vi "Main.vi"() -> ()   [LabVIEW 2020]
uses:
  _lib/Root.lvlibp/Root.lvclass
  0c08c685-3369-46e5-9f6c-9a8c11b7282d.vi
  0c08c685-3369-46e5-9f6c-9a8c11b7282d.vi/a06a5617-693f-4e7a-880a-01e7210d5b34.vi
  0c08c685-3369-46e5-9f6c-9a8c11b7282d.vi/a86dd2ad-e02c-4951-b0d8-e9482f107a59.vi
  0c08c685-3369-46e5-9f6c-9a8c11b7282d.vi/2fe82b45-d63b-4374-a5d2-02a331a98b71.vi
  0c08c685-3369-46e5-9f6c-9a8c11b7282d.vi/09bee0a5-df0d-4391-90c9-116df187134d.vi
  0c08c685-3369-46e5-9f6c-9a8c11b7282d.vi/1c1c90a5-34b6-4f03-abf8-3ec97f905fca.vi
  0c08c685-3369-46e5-9f6c-9a8c11b7282d.vi/c25736fa-ea5e-462f-8a61-d5812afa17aa.vi
  <userlib>/_NEVSTOP/LabVIEW-ClassProviderShell/_Support/__File Exists - Scalar__ogtk.vi
  <userlib>/_NEVSTOP/LabVIEW-ClassProviderShell/_Support/__Strip Path Extension - String__ogtk.vi
  <vilib>/Utility/LVLibp/Get Exported File List.vi
  <vilib>/Utility/LVClass/Get LV Class Default Value.vi
  <userlib>/_NEVSTOP/LabVIEW-ClassProviderShell/_Support/__Wait(ms) If Input Valid.vi
  <vilib>/Utility/libraryn.llb/Recursive File List.vi
  <vilib>/Utility/libraryn.llb/Check if File or Folder Exists.vi
  <userlib>/_NEVSTOP/LabVIEW-ClassProviderShell/_Support/__Recursive File List with Exclude Option.vi
panel:
  out "result":dbl
  in  "b":dbl=20.0
  in  "a":dbl=100.0
  in  "Listbox":i32(listbox)
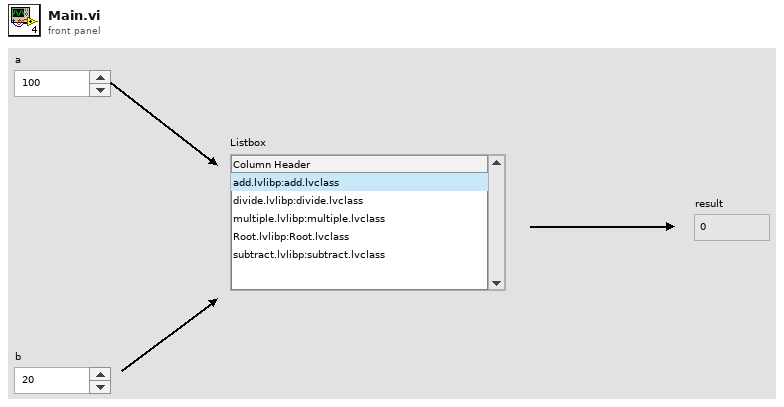
[diagram p1: front panel]
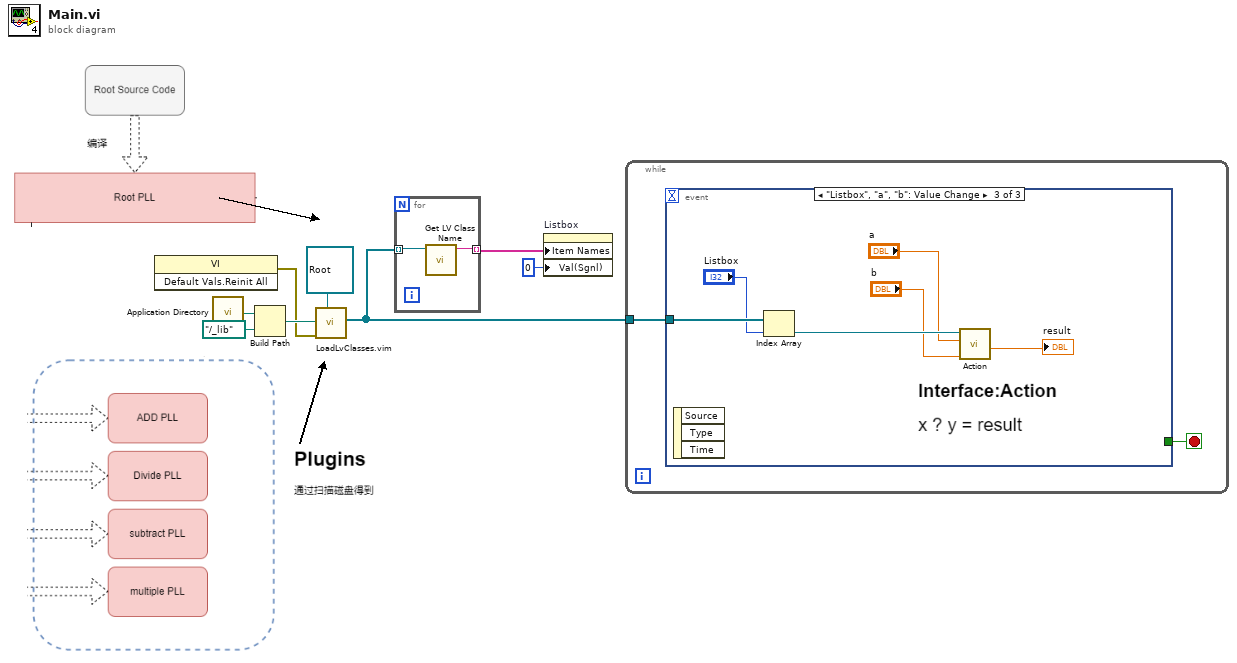
[diagram p0: block diagram]
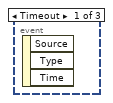
[diagram p2: hidden frame]
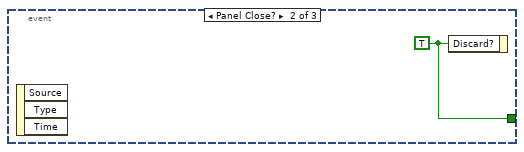
[diagram p3: hidden frame]
diagram:
  n1 = invoke class="VI" method="Default Vals.Reinit All"() -> (error out=w1:errorcluster)  [unwired: 3 in, 2 out]
  n2 = call <vilib>:"Application Directory.vi"() -> ("Application Directory"=w7:path)
  n3 = Build Path(base path=w7, name or relative path=path "../_lib") -> (appended path=w5:path)
  n4 = call "LoadLvClasses.vim"("ClassType"=refnum<class "Root.lvclass"> refnum ("Root.lvlibp:Root.lvclass"), "error in (no error)"=w1, "Path"=w5) -> ("Loaded Classes"=w4:refnum<class "Root.lvclass">[])  [unwired: 7 in, 1 out]
  n5 = for {
    tunnel: w4 -> [w10] mode=indexing
    tunnel: [w9] -> w3 mode=indexing
    n6 = call <vilib>:"Get LV Class Name.vi"("object"=w10) -> ("class name"=w9:string)  [unwired: 9 in, 1 out]
  }
  n7 = property on="Listbox" class="LstBox (strict)"("Item Names"=w3, "Val(Sgnl)"=0 ("Listbox")) -> ()  [unwired: 2 in, 2 out]
  n8 = while {
    tunnel: w4 -> [w11]
    stop <- w12 stop-if-true
    n9 = event shown="[2] \"Listbox\", \"a\", \"b\": Value Change" {
      selector: _ -> [_ _ _]
      dyn-events: _ -> [_ _ _]
      timeout: _ -> [_ _ _]
      tunnel: [_ w13 _] -> w12
      tunnel: w11 -> [_ _ w19]
      event Timeout {
        n10 = event-data() -> ()  [unwired: 1 in, 3 out]
      }
      event Panel Close? {
        w13 = TRUE ("Discard?")
        n11 = event-data() -> ()  [unwired: 1 in, 3 out]
        n12 = event-data("Discard?"=w13) -> ()  [unwired: 1 in, 1 out]
      }
      event "Listbox", "a", "b": Value Change {
        n13 = event-data() -> ()  [unwired: 1 in, 3 out]
        n14 = Index Array(array=w19, index="Listbox") -> (element=w17:refnum<class "Root.lvclass">)
        n15 = call-dynamic "Action.vi"("b"="b", "a"="a", "Root in"=w17) -> ("result"=→"result":dbl)  [unwired: 7 in, 1 out]
      }
    }
  }
